vi "Write Homing.vi"(8 "error in (no error)":errorcluster, 10 "Homing":variant, 11 "FW Arduino Control in":refnum<class "FW Arduino Control.lvclass">) -> (0 "error out":errorcluster, 3 "FW Arduino Control out":refnum<class "FW Arduino Control.lvclass">)   [LabVIEW 2021, in "FW Arduino Control.lvclass"]
uses:
  FW Arduino Control.lvclass
  Filter Wheel Arduino Homing cluster.ctl
  FW Arduino Control.lvclass/FW Arduino Control.ctl
  Filter Wheel Object/Filter Wheel.lvclass
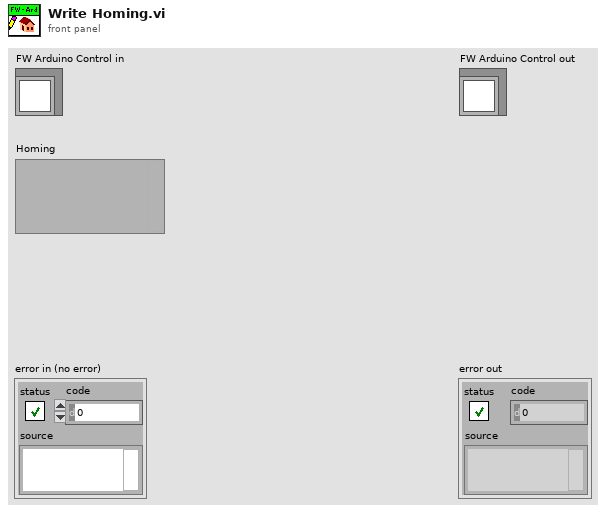
[diagram p1: front panel]
types:
  T1 = typedef "Filter Wheel Arduino Homing cluster.ctl" = cluster{"Direction (F: CW)":bool, "Speed":i32, "Accel":i32, "Min Distance":i32, "Short Leg":i32, "Error Cnts":i32}
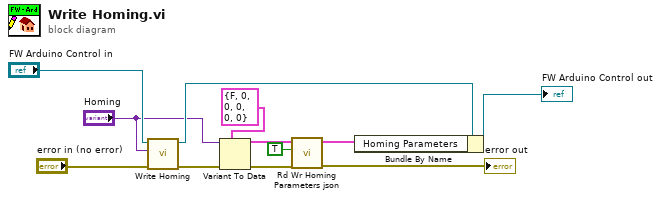
[diagram p0: block diagram]
diagram:
  n1 = call-parent "Write Homing.vi"("error in (no error)"="error in (no error)", "Homing"="Homing", "Filter Wheel in"="FW Arduino Control in") -> ("error out"=w8:errorcluster, "Filter Wheel out"=w10:refnum<class "FW Arduino Control.lvclass">)  [unwired: 7 in]
  n2 = Variant To Data(error in=w8, type=T1 {"Direction (F: CW)"=FALSE, "Speed"=0, "Accel"=0, "Min Distance"=0, "Short Leg"=0, "Error Cnts"=0} ("Homing Parameters"), Variant="Homing") -> (data=w3:T1, error out=w5:errorcluster)
  n3 = call "Rd Wr Homing Parameters json.vi"("error in (no error)"=w5, "Write? (F:Read)"=TRUE, "Homing Parameters"=w3) -> ("error out"=→"error out":errorcluster, "Homing Parameters"=w1:T1)  [unwired: 7 in]
  n4 = Bundle By Name(cluster=w10, "Homing Parameters"=w1) -> (→"FW Arduino Control out":refnum<class "FW Arduino Control.lvclass">)
